vi "LINX - Servo 1 Channel and Analog Read.vi"() -> ()   [LabVIEW 2016]
doc: "This example demonstrates how to control a servo using LINX."
uses:
  <vilib>/MakerHub/LINX/Public/Peripherals/Analog/Analog Read 1 Chan.vi
  <vilib>/MakerHub/LINX/Public/Peripherals/Analog/Analog Read N Chans.vi
  <vilib>/MakerHub/LINX/Private/Local IO/LinxAnalogRead.vi
  <vilib>/MakerHub/LINX/Public/Utilities/Check Channel.vi
  <vilib>/MakerHub/LINX/Public/Utilities/Open Serial.vi
  <vilib>/MakerHub/LINX/Public/Sensors/Motion/Servo/Servo Open One Channel.vi
  <vilib>/MakerHub/LINX/Public/Sensors/Motion/Servo/Servo Set Pulse Width One Channel.vi
  <vilib>/MakerHub/LINX/Private/Utilties/Generate Error.vi
  <vilib>/MakerHub/LINX/Public/Sensors/Motion/Servo/Servo Close One Channel.vi
  <vilib>/MakerHub/LINX/LMH-LINX.lvlib
  <vilib>/MakerHub/LINX/Public/Sensors/Motion/Servo/Servo.lvlib
panel:
  out "Analog Data":dbl(graph)
  in  "AI Channel":u8
  out "Loop Rate (Hz)":u32
  in  "Servo Position":u16(knob)=1493 scale=500.0..2500.0
  in  "Servo Channel":u8=2
  in  "Stop Button":bool
  in  "Serial Port":refnum<visa-resource-name>
  # "Servo Example (Serial Interface)\n\nThis example demonstrates how to control a servo.\n\nInstructions\n1. Select the COM Port associated with the LINX Device.\n2. Select the Servo Channel connected to the servo to control.\n3. Click the Run Arrow.\n4. Adjust the dial to control the digital pulse width sent to the servo.  The pulse \n    width determines the servo position.  A 1500 uS pulse is typically 90 degrees.  \n    The maximum angle will depend on the sepcific servo used."
  # "Servo Position \n(Pulse Width uS)"
  # "LINX Device Settings"
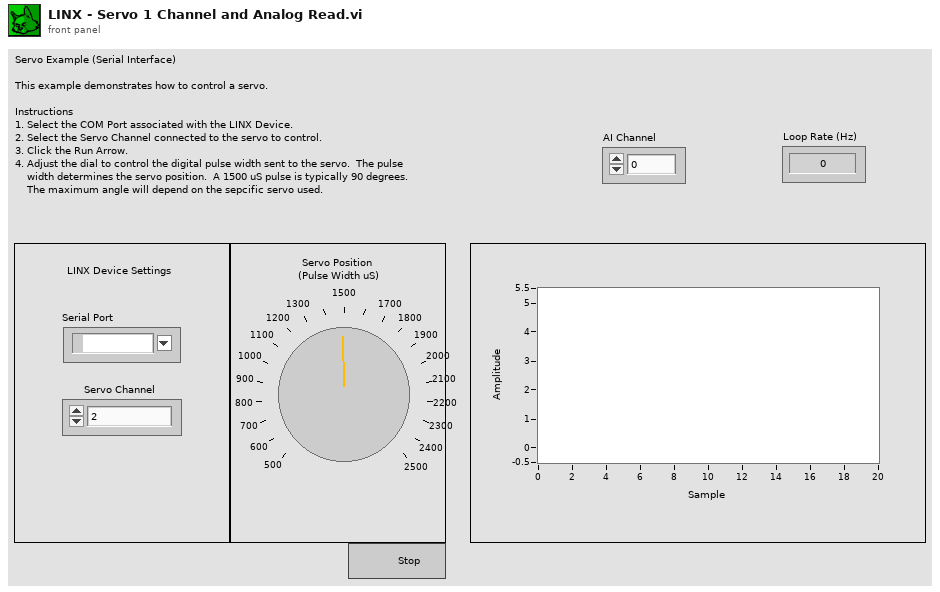
[diagram p1: front panel]
types:
  T1 = typedef "LMH-LINX.lvlib/LINX Ref.ctl" = cluster{"IO":T2, "Interface":T3, "LINX Device Config":T4}
  T2 = typedef "LMH-LINX.lvlib/Platform.ctl" = enum16{"Remote", "Local"}
  T3 = typedef "LMH-LINX.lvlib/Interface.ctl" = enum16{"Serial", "TCP"}
  T4 = typedef "LMH-LINX.lvlib/Device.lvlib/LINX Device Config.ctl" = cluster{"Interface":T3, "COM Port":refnum<visa-resource-name>, "TCP Configuration":T5, "Device Family":u8, "Device ID":u8, "Device Name":string, "TCP Ref":refnum<k5>, "Channels":T6}
  T5 = typedef "LMH-LINX.lvlib/Device.lvlib/TCP Config.ctl" = cluster{"IP Address":string, "Port":u16}
  T6 = typedef "LMH-LINX.lvlib/Channels.ctl" = cluster{"DI":u8[], "DO":u8[], "AI":u8[], "AO":u8[], "PWM":u8[], "QE":u8[], "UART":u8[], "I2C 2":u8[], "SPI":u8[], "CAN":u8[], "Servo":u8[], "AI Ref (V)":dbl, "AI Resolution (Bits)":u8, "AO Ref (V)":dbl, "AO Resolution (Bits)":u8}
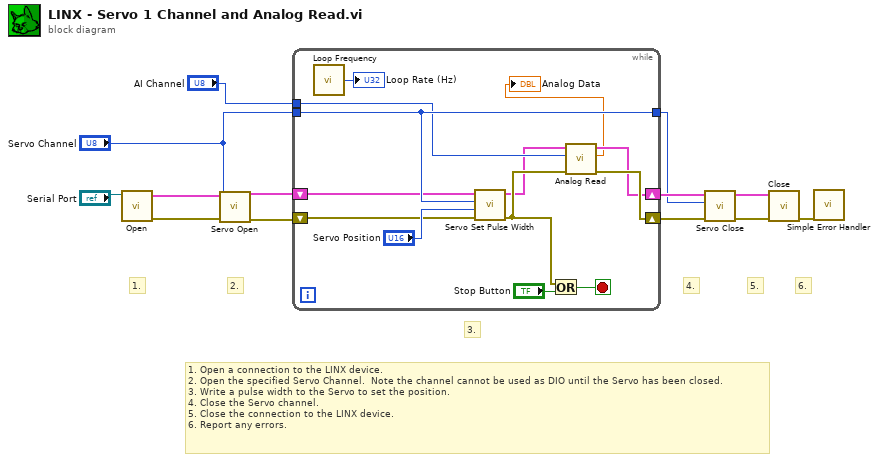
[diagram p0: block diagram]
diagram:
  # "6."
  # "1. Open a connection to the LINX device.\n2. Open the specified Servo Channel.  Note the channel cannot be used as DIO until the Servo has been closed.\n3. Write a pulse width to the Servo to set the position.\n4. Close the Servo channel.  \n5. Close the connection to the LINX device.\n6. Report any errors."
  # "5."
  # "4."
  # "3."
  # "2."
  # "1."
  n1 = call-poly <vilib>:"Open.vi"("Serial Port"="Serial Port") -> ("Error Out"=w12:errorcluster, "LINX Resource"=w11:T1)  [unwired: 8 in, 1 out]
  n2 = call-poly <vilib>:"Servo Open.vi"("Error In"=w12, "Servo Channel"="Servo Channel", "LINX Resource"=w11) -> ("Error Out"=w10:errorcluster, "LINX Resource"=w9:T1)  [unwired: 7 in]
  n3 = while {
    shift-right: [w18] -> w3
    shift-left: w10 -> [w20]
    tunnel: "Servo Channel" -> [w23]
    shift-right: [w15] -> w6
    shift-left: w9 -> [w21]
    tunnel: [w23] -> w2
    tunnel: "AI Channel" -> [w17]
    stop <- w26 stop-if-true
    n4 = call <vilib>:"Loop Frequency.vi"() -> ("Loop Rate (Hz)"=→"Loop Rate (Hz)":u32)
    n5 = call-poly <vilib>:"Servo Set Pulse Width.vi"("Error In"=w20, "Pulse Width (uS)"="Servo Position", "Servo Channel"=w23, "LINX Resource"=w21) -> ("Error Out"=w19:errorcluster, "LINX Resource"=w16:T1)  [unwired: 6 in]
    n6 = Or(x=w19, y="Stop Button") -> (x .or. y?=w26:bool)
    n7 = call-poly <vilib>:"Analog Read.vi"("Error In"=w19, "Analog Channel"=w17, "LINX Resource"=w16) -> ("Error Out"=w18:errorcluster, "Voltage"=→"Analog Data":dbl, "LINX Resource"=w15:T1)  [unwired: 5 in, 1 out]
  }
  n8 = call-poly <vilib>:"Servo Close.vi"("Error In"=w3, "Servo Channel"=w2, "LINX Resource"=w6) -> ("Error Out"=w4:errorcluster, "LINX Resource"=w5:T1)  [unwired: 7 in]
  n9 = call <vilib>:"Close.vi"("Error In"=w4, "LINX Resource"=w5) -> ("Error Out"=w7:errorcluster)  [unwired: 9 in]
  n10 = call <vilib>:"Simple Error Handler.vi"("error in (no error)"=w7) -> ()  [unwired: 4 in, 5 out]
